vi "StringToCoreArray.vi"(11 "Error In":errorcluster) -> (4 "Key Value Variant":variant, 15 "Error Out":errorcluster)   [LabVIEW 2016, in "Drona.lvlib" / "KeyboardSimulation.lvlib"]
doc: "Gives the key value pair variant output, for various letters present in keyboard"
uses:
  KeyboardSimulation.lvlib
  typedef/VirtualKey.ctl
  typedef/Action.ctl
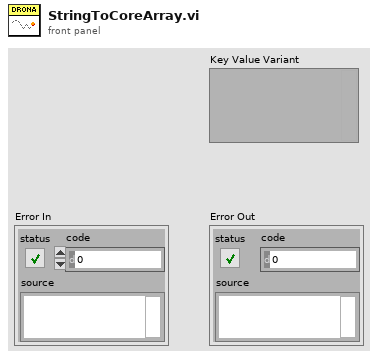
[diagram p1: front panel]
types:
  T1 = typedef "Drona.lvlib/KeyboardSimulation.lvlib/VirtualKey.ctl" = u8
  T2 = typedef "Drona.lvlib/KeyboardSimulation.lvlib/Action.ctl" = enum16{"Press", "Up", "Down"}
  T3 = cluster{"Key":T1, "Action":T2, "Delay (ms)":u32}[]
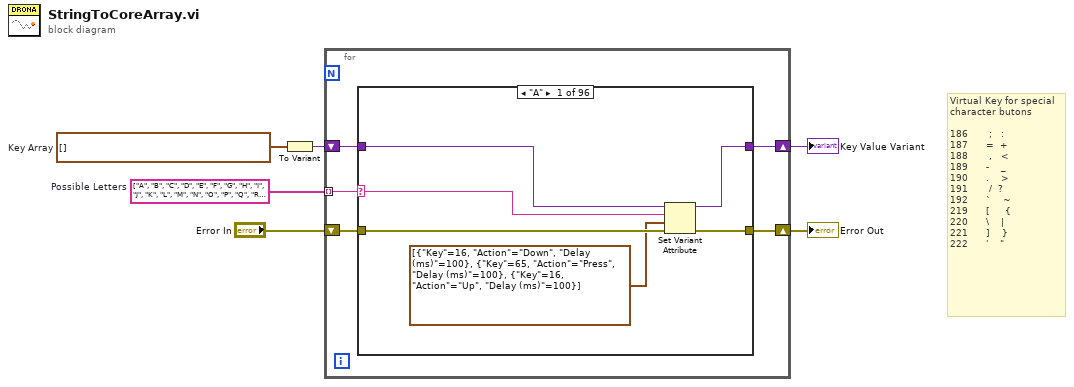
[diagram p0: block diagram]
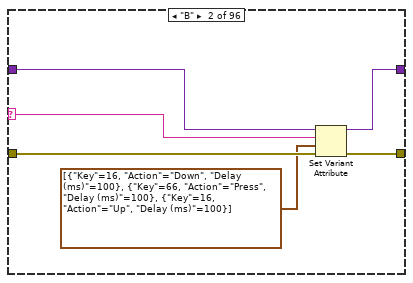
[diagram p2: hidden frame]
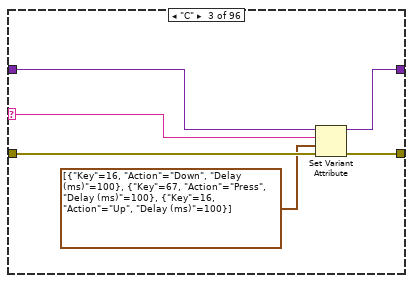
[diagram p3: hidden frame]
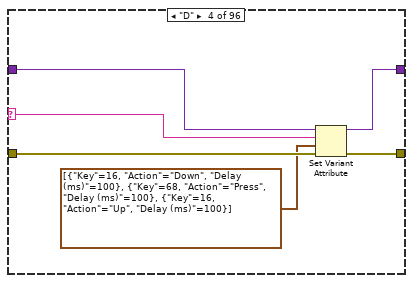
[diagram p4: hidden frame]
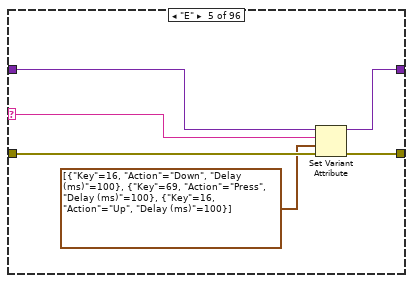
[diagram p5: hidden frame]
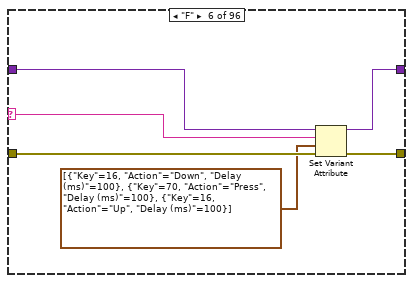
[diagram p6: hidden frame]
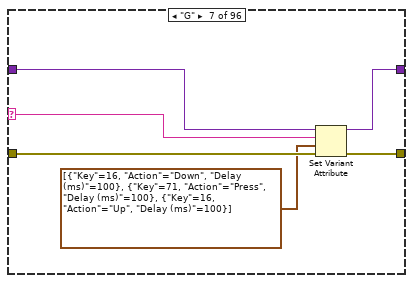
[diagram p7: hidden frame]
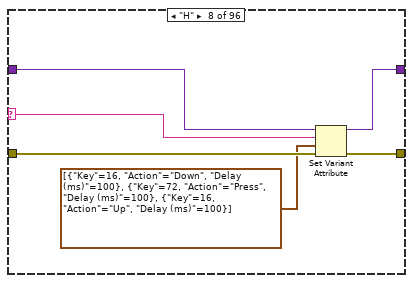
[diagram p8: hidden frame]
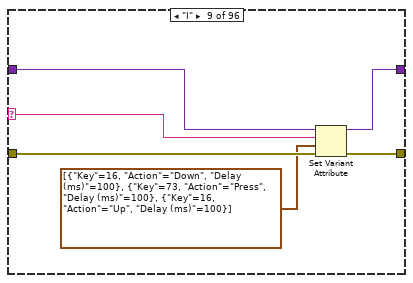
[diagram p9: hidden frame]
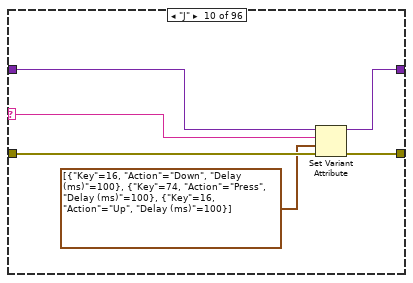
[diagram p10: hidden frame]
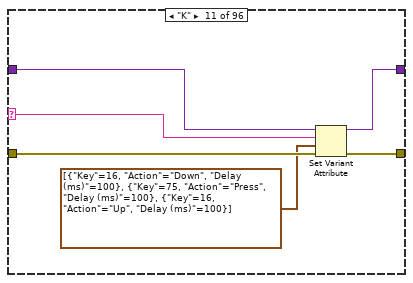
[diagram p11: hidden frame]
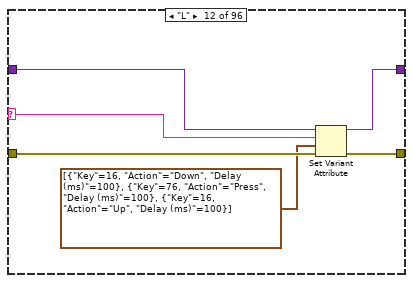
[diagram p12: hidden frame]
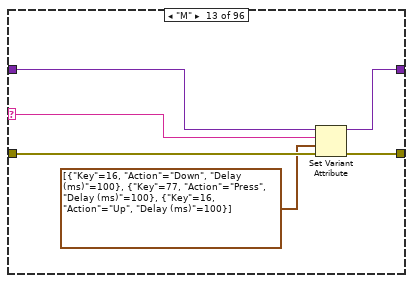
[diagram p13: hidden frame]
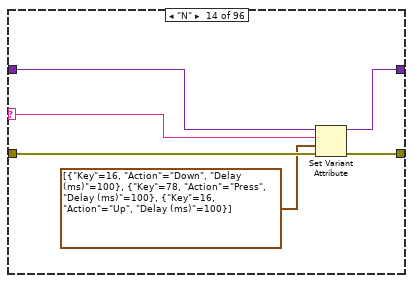
[diagram p14: hidden frame]
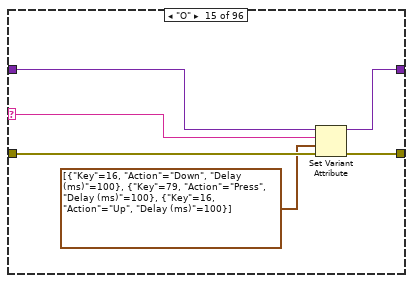
[diagram p15: hidden frame]
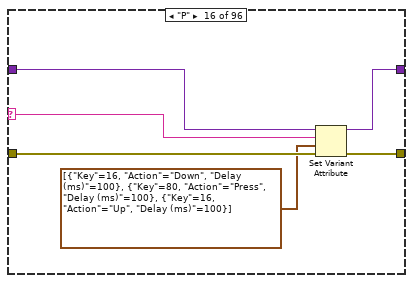
[diagram p16: hidden frame]
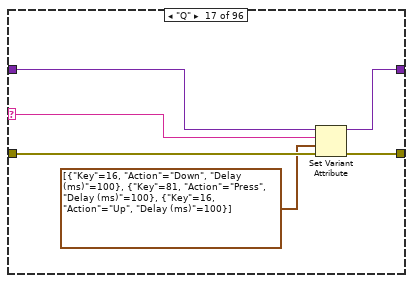
[diagram p17: hidden frame]
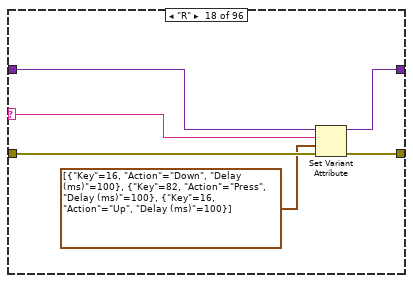
[diagram p18: hidden frame]
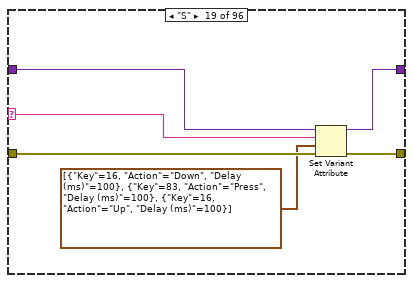
[diagram p19: hidden frame]
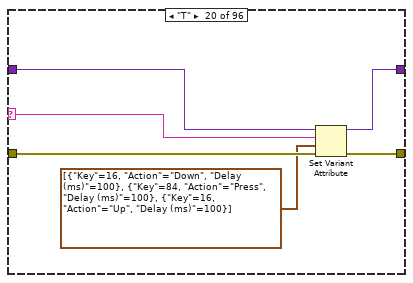
[diagram p20: hidden frame]
diagram:
  w4 = T3 []  # Key Array
  w5 = string[] ["A", "B", "C", "D", "E", "F", "G", "H", "I", "J", "K", "L", "M", "N", "O", "P", "Q", "R", "S", "T", "U", "V", "W", "X", "Y", "Z", "a", "b", "c", "d", "e", "f", "g", "h", "i", "j", "k", "l", "m", "n", "o", "p", "q", "r", "s", "t", "u", "v", "w", "x", "y", "z", "1", "2", "3", "4", "5", "6", "7", "8", "9", "0", "!", "@", "#", "$", "%", "^", "&", "*", "(", ")", ";", ":", "=", "+", ",", "<", "-", "_", ".", ">", "/", "?", "`", "~", "[", "{", "Back Slash", "|", "]", "}", "Single Quotes", "Double Quotes", "Space"]  # Possible Letters
  # "Virtual Key for special character butons\n\n186       ;   :\n187      =  +\n188       ,   <\n189      -    _\n190      .    >\n191       /  ?\n192      `    ~\n219      [     {\n220      \\    |\n221      ]    }\n222      '    \""
  n1 = To Variant(anything=w4) -> (Variant=w3:variant)
  n2 = for {
    shift-right: [w7] -> w1
    shift-left: w3 -> [w9]
    shift-right: [w8] -> w2
    shift-left: "Error In" -> [w10]
    tunnel: w5 -> [w11] mode=indexing
    n3 = case shown="\"A\"" w11 {
      selector: w11 -> [w15 w21 w27 w33 w39 w45 w51 w57 w63 w69 w75 w81 w87 w93 w99 w105 w111 w117 w123 w129 w135 w141 w147 w153 w159 w165 w171 w177 w183 w189 w195 w201 w207 w213 w219 w225 w231 w237 w243 w249 w255 w261 w267 w273 w279 w285 w291 w297 w303 w309 w315 w321 w327 w333 w339 w345 w351 w357 w363 w369 w375 w381 w387 w393 w399 w405 w411 w417 w423 w429 w435 w441 w447 w453 w459 w465 w471 w477 w483 w489 w495 w501 w507 w513 w519 w525 w531 w537 _ w549 w555 w561 _ _ _ _]
      tunnel: w10 -> [w17 w23 w29 w35 w41 w47 w53 w59 w65 w71 w77 w83 w89 w95 w101 w107 w113 w119 w125 w131 w137 w143 w149 w155 w161 w167 w173 w179 w185 w191 w197 w203 w209 w215 w221 w227 w233 w239 w245 w251 w257 w263 w269 w275 w281 w287 w293 w299 w305 w311 w317 w323 w329 w335 w341 w347 w353 w359 w365 w371 w377 w383 w389 w395 w401 w407 w413 w419 w425 w431 w437 w443 w449 w455 w461 w467 w473 w479 w485 w491 w497 w503 w509 w515 w521 w527 w533 w539 w545 w551 w557 w563 w569 w575 w581 w582]
      tunnel: w9 -> [w16 w22 w28 w34 w40 w46 w52 w58 w64 w70 w76 w82 w88 w94 w100 w106 w112 w118 w124 w130 w136 w142 w148 w154 w160 w166 w172 w178 w184 w190 w196 w202 w208 w214 w220 w226 w232 w238 w244 w250 w256 w262 w268 w274 w280 w286 w292 w298 w304 w310 w316 w322 w328 w334 w340 w346 w352 w358 w364 w370 w376 w382 w388 w394 w400 w406 w412 w418 w424 w430 w436 w442 w448 w454 w460 w466 w472 w478 w484 w490 w496 w502 w508 w514 w520 w526 w532 w538 w544 w550 w556 w562 w568 w574 w580 w583]
      tunnel: [w14 w20 w26 w32 w38 w44 w50 w56 w62 w68 w74 w80 w86 w92 w98 w104 w110 w116 w122 w128 w134 w140 w146 w152 w158 w164 w170 w176 w182 w188 w194 w200 w206 w212 w218 w224 w230 w236 w242 w248 w254 w260 w266 w272 w278 w284 w290 w296 w302 w308 w314 w320 w326 w332 w338 w344 w350 w356 w362 w368 w374 w380 w386 w392 w398 w404 w410 w416 w422 w428 w434 w440 w446 w452 w458 w464 w470 w476 w482 w488 w494 w500 w506 w512 w518 w524 w530 w536 w543 w548 w554 w560 w567 w573 w579 w582] -> w8
      tunnel: [w13 w19 w25 w31 w37 w43 w49 w55 w61 w67 w73 w79 w85 w91 w97 w103 w109 w115 w121 w127 w133 w139 w145 w151 w157 w163 w169 w175 w181 w187 w193 w199 w205 w211 w217 w223 w229 w235 w241 w247 w253 w259 w265 w271 w277 w283 w289 w295 w301 w307 w313 w319 w325 w331 w337 w343 w349 w355 w361 w367 w373 w379 w385 w391 w397 w403 w409 w415 w421 w427 w433 w439 w445 w451 w457 w463 w469 w475 w481 w487 w493 w499 w505 w511 w517 w523 w529 w535 w542 w547 w553 w559 w566 w572 w578 w583] -> w7
      frame "A" {
        n4 = Set Variant Attribute(Variant=w16, name=w15, value=T3 [{"Key"=16, "Action"=enum."Down", "Delay (ms)"=100}, {"Key"=65, "Action"=enum."Press", "Delay (ms)"=100}, {"Key"=16, "Action"=enum."Up", "Delay (ms)"=100}] ("Key Array"), error in=w17) -> (Variant out=w13:variant, error out=w14:errorcluster)  [unwired: 1 out]
      }
      frame "B" {
        n5 = Set Variant Attribute(Variant=w22, name=w21, value=T3 [{"Key"=16, "Action"=enum."Down", "Delay (ms)"=100}, {"Key"=66, "Action"=enum."Press", "Delay (ms)"=100}, {"Key"=16, "Action"=enum."Up", "Delay (ms)"=100}] ("Key Array"), error in=w23) -> (Variant out=w19:variant, error out=w20:errorcluster)  [unwired: 1 out]
      }
      frame "C" {
        n6 = Set Variant Attribute(Variant=w28, name=w27, value=T3 [{"Key"=16, "Action"=enum."Down", "Delay (ms)"=100}, {"Key"=67, "Action"=enum."Press", "Delay (ms)"=100}, {"Key"=16, "Action"=enum."Up", "Delay (ms)"=100}] ("Key Array"), error in=w29) -> (Variant out=w25:variant, error out=w26:errorcluster)  [unwired: 1 out]
      }
      frame "D" {
        n7 = Set Variant Attribute(Variant=w34, name=w33, value=T3 [{"Key"=16, "Action"=enum."Down", "Delay (ms)"=100}, {"Key"=68, "Action"=enum."Press", "Delay (ms)"=100}, {"Key"=16, "Action"=enum."Up", "Delay (ms)"=100}] ("Key Array"), error in=w35) -> (Variant out=w31:variant, error out=w32:errorcluster)  [unwired: 1 out]
      }
      frame "E" {
        n8 = Set Variant Attribute(Variant=w40, name=w39, value=T3 [{"Key"=16, "Action"=enum."Down", "Delay (ms)"=100}, {"Key"=69, "Action"=enum."Press", "Delay (ms)"=100}, {"Key"=16, "Action"=enum."Up", "Delay (ms)"=100}] ("Key Array"), error in=w41) -> (Variant out=w37:variant, error out=w38:errorcluster)  [unwired: 1 out]
      }
      frame "F" {
        n9 = Set Variant Attribute(Variant=w46, name=w45, value=T3 [{"Key"=16, "Action"=enum."Down", "Delay (ms)"=100}, {"Key"=70, "Action"=enum."Press", "Delay (ms)"=100}, {"Key"=16, "Action"=enum."Up", "Delay (ms)"=100}] ("Key Array"), error in=w47) -> (Variant out=w43:variant, error out=w44:errorcluster)  [unwired: 1 out]
      }
      frame "G" {
        n10 = Set Variant Attribute(Variant=w52, name=w51, value=T3 [{"Key"=16, "Action"=enum."Down", "Delay (ms)"=100}, {"Key"=71, "Action"=enum."Press", "Delay (ms)"=100}, {"Key"=16, "Action"=enum."Up", "Delay (ms)"=100}] ("Key Array"), error in=w53) -> (Variant out=w49:variant, error out=w50:errorcluster)  [unwired: 1 out]
      }
      frame "H" {
        n11 = Set Variant Attribute(Variant=w58, name=w57, value=T3 [{"Key"=16, "Action"=enum."Down", "Delay (ms)"=100}, {"Key"=72, "Action"=enum."Press", "Delay (ms)"=100}, {"Key"=16, "Action"=enum."Up", "Delay (ms)"=100}] ("Key Array"), error in=w59) -> (Variant out=w55:variant, error out=w56:errorcluster)  [unwired: 1 out]
      }
      frame "I" {
        n12 = Set Variant Attribute(Variant=w64, name=w63, value=T3 [{"Key"=16, "Action"=enum."Down", "Delay (ms)"=100}, {"Key"=73, "Action"=enum."Press", "Delay (ms)"=100}, {"Key"=16, "Action"=enum."Up", "Delay (ms)"=100}] ("Key Array"), error in=w65) -> (Variant out=w61:variant, error out=w62:errorcluster)  [unwired: 1 out]
      }
      frame "J" {
        n13 = Set Variant Attribute(Variant=w70, name=w69, value=T3 [{"Key"=16, "Action"=enum."Down", "Delay (ms)"=100}, {"Key"=74, "Action"=enum."Press", "Delay (ms)"=100}, {"Key"=16, "Action"=enum."Up", "Delay (ms)"=100}] ("Key Array"), error in=w71) -> (Variant out=w67:variant, error out=w68:errorcluster)  [unwired: 1 out]
      }
      frame "K" {
        n14 = Set Variant Attribute(Variant=w76, name=w75, value=T3 [{"Key"=16, "Action"=enum."Down", "Delay (ms)"=100}, {"Key"=75, "Action"=enum."Press", "Delay (ms)"=100}, {"Key"=16, "Action"=enum."Up", "Delay (ms)"=100}] ("Key Array"), error in=w77) -> (Variant out=w73:variant, error out=w74:errorcluster)  [unwired: 1 out]
      }
      frame "L" {
        n15 = Set Variant Attribute(Variant=w82, name=w81, value=T3 [{"Key"=16, "Action"=enum."Down", "Delay (ms)"=100}, {"Key"=76, "Action"=enum."Press", "Delay (ms)"=100}, {"Key"=16, "Action"=enum."Up", "Delay (ms)"=100}] ("Key Array"), error in=w83) -> (Variant out=w79:variant, error out=w80:errorcluster)  [unwired: 1 out]
      }
      frame "M" {
        n16 = Set Variant Attribute(Variant=w88, name=w87, value=T3 [{"Key"=16, "Action"=enum."Down", "Delay (ms)"=100}, {"Key"=77, "Action"=enum."Press", "Delay (ms)"=100}, {"Key"=16, "Action"=enum."Up", "Delay (ms)"=100}] ("Key Array"), error in=w89) -> (Variant out=w85:variant, error out=w86:errorcluster)  [unwired: 1 out]
      }
      frame "N" {
        n17 = Set Variant Attribute(Variant=w94, name=w93, value=T3 [{"Key"=16, "Action"=enum."Down", "Delay (ms)"=100}, {"Key"=78, "Action"=enum."Press", "Delay (ms)"=100}, {"Key"=16, "Action"=enum."Up", "Delay (ms)"=100}] ("Key Array"), error in=w95) -> (Variant out=w91:variant, error out=w92:errorcluster)  [unwired: 1 out]
      }
      frame "O" {
        n18 = Set Variant Attribute(Variant=w100, name=w99, value=T3 [{"Key"=16, "Action"=enum."Down", "Delay (ms)"=100}, {"Key"=79, "Action"=enum."Press", "Delay (ms)"=100}, {"Key"=16, "Action"=enum."Up", "Delay (ms)"=100}] ("Key Array"), error in=w101) -> (Variant out=w97:variant, error out=w98:errorcluster)  [unwired: 1 out]
      }
      frame "P" {
        n19 = Set Variant Attribute(Variant=w106, name=w105, value=T3 [{"Key"=16, "Action"=enum."Down", "Delay (ms)"=100}, {"Key"=80, "Action"=enum."Press", "Delay (ms)"=100}, {"Key"=16, "Action"=enum."Up", "Delay (ms)"=100}] ("Key Array"), error in=w107) -> (Variant out=w103:variant, error out=w104:errorcluster)  [unwired: 1 out]
      }
      frame "Q" {
        n20 = Set Variant Attribute(Variant=w112, name=w111, value=T3 [{"Key"=16, "Action"=enum."Down", "Delay (ms)"=100}, {"Key"=81, "Action"=enum."Press", "Delay (ms)"=100}, {"Key"=16, "Action"=enum."Up", "Delay (ms)"=100}] ("Key Array"), error in=w113) -> (Variant out=w109:variant, error out=w110:errorcluster)  [unwired: 1 out]
      }
      frame "R" {
        n21 = Set Variant Attribute(Variant=w118, name=w117, value=T3 [{"Key"=16, "Action"=enum."Down", "Delay (ms)"=100}, {"Key"=82, "Action"=enum."Press", "Delay (ms)"=100}, {"Key"=16, "Action"=enum."Up", "Delay (ms)"=100}] ("Key Array"), error in=w119) -> (Variant out=w115:variant, error out=w116:errorcluster)  [unwired: 1 out]
      }
      frame "S" {
        n22 = Set Variant Attribute(Variant=w124, name=w123, value=T3 [{"Key"=16, "Action"=enum."Down", "Delay (ms)"=100}, {"Key"=83, "Action"=enum."Press", "Delay (ms)"=100}, {"Key"=16, "Action"=enum."Up", "Delay (ms)"=100}] ("Key Array"), error in=w125) -> (Variant out=w121:variant, error out=w122:errorcluster)  [unwired: 1 out]
      }
      frame "T" {
        n23 = Set Variant Attribute(Variant=w130, name=w129, value=T3 [{"Key"=16, "Action"=enum."Down", "Delay (ms)"=100}, {"Key"=84, "Action"=enum."Press", "Delay (ms)"=100}, {"Key"=16, "Action"=enum."Up", "Delay (ms)"=100}] ("Key Array"), error in=w131) -> (Variant out=w127:variant, error out=w128:errorcluster)  [unwired: 1 out]
      }
      frame "U" {
        n24 = Set Variant Attribute(Variant=w136, name=w135, value=T3 [{"Key"=16, "Action"=enum."Down", "Delay (ms)"=100}, {"Key"=85, "Action"=enum."Press", "Delay (ms)"=100}, {"Key"=16, "Action"=enum."Up", "Delay (ms)"=100}] ("Key Array"), error in=w137) -> (Variant out=w133:variant, error out=w134:errorcluster)  [unwired: 1 out]
      }
      frame "V" {
        n25 = Set Variant Attribute(Variant=w142, name=w141, value=T3 [{"Key"=16, "Action"=enum."Down", "Delay (ms)"=100}, {"Key"=86, "Action"=enum."Press", "Delay (ms)"=100}, {"Key"=16, "Action"=enum."Up", "Delay (ms)"=100}] ("Key Array"), error in=w143) -> (Variant out=w139:variant, error out=w140:errorcluster)  [unwired: 1 out]
      }
      frame "W" {
        n26 = Set Variant Attribute(Variant=w148, name=w147, value=T3 [{"Key"=16, "Action"=enum."Down", "Delay (ms)"=100}, {"Key"=87, "Action"=enum."Press", "Delay (ms)"=100}, {"Key"=16, "Action"=enum."Up", "Delay (ms)"=100}] ("Key Array"), error in=w149) -> (Variant out=w145:variant, error out=w146:errorcluster)  [unwired: 1 out]
      }
      frame "X" {
        n27 = Set Variant Attribute(Variant=w154, name=w153, value=T3 [{"Key"=16, "Action"=enum."Down", "Delay (ms)"=100}, {"Key"=88, "Action"=enum."Press", "Delay (ms)"=100}, {"Key"=16, "Action"=enum."Up", "Delay (ms)"=100}] ("Key Array"), error in=w155) -> (Variant out=w151:variant, error out=w152:errorcluster)  [unwired: 1 out]
      }
      frame "Y" {
        n28 = Set Variant Attribute(Variant=w160, name=w159, value=T3 [{"Key"=16, "Action"=enum."Down", "Delay (ms)"=100}, {"Key"=89, "Action"=enum."Press", "Delay (ms)"=100}, {"Key"=16, "Action"=enum."Up", "Delay (ms)"=100}] ("Key Array"), error in=w161) -> (Variant out=w157:variant, error out=w158:errorcluster)  [unwired: 1 out]
      }
      frame "Z" {
        n29 = Set Variant Attribute(Variant=w166, name=w165, value=T3 [{"Key"=16, "Action"=enum."Down", "Delay (ms)"=100}, {"Key"=90, "Action"=enum."Press", "Delay (ms)"=100}, {"Key"=16, "Action"=enum."Up", "Delay (ms)"=100}] ("Key Array"), error in=w167) -> (Variant out=w163:variant, error out=w164:errorcluster)  [unwired: 1 out]
      }
      frame "a" {
        n30 = Set Variant Attribute(Variant=w172, name=w171, value=T3 [{"Key"=65, "Action"=enum."Press", "Delay (ms)"=100}] ("Key Array"), error in=w173) -> (Variant out=w169:variant, error out=w170:errorcluster)  [unwired: 1 out]
      }
      frame "b" {
        n31 = Set Variant Attribute(Variant=w178, name=w177, value=T3 [{"Key"=66, "Action"=enum."Press", "Delay (ms)"=100}] ("Key Array"), error in=w179) -> (Variant out=w175:variant, error out=w176:errorcluster)  [unwired: 1 out]
      }
      frame "c" {
        n32 = Set Variant Attribute(Variant=w184, name=w183, value=T3 [{"Key"=67, "Action"=enum."Press", "Delay (ms)"=100}] ("Key Array"), error in=w185) -> (Variant out=w181:variant, error out=w182:errorcluster)  [unwired: 1 out]
      }
      frame "d" {
        n33 = Set Variant Attribute(Variant=w190, name=w189, value=T3 [{"Key"=68, "Action"=enum."Press", "Delay (ms)"=100}] ("Key Array"), error in=w191) -> (Variant out=w187:variant, error out=w188:errorcluster)  [unwired: 1 out]
      }
      frame "e" {
        n34 = Set Variant Attribute(Variant=w196, name=w195, value=T3 [{"Key"=69, "Action"=enum."Press", "Delay (ms)"=100}] ("Key Array"), error in=w197) -> (Variant out=w193:variant, error out=w194:errorcluster)  [unwired: 1 out]
      }
      frame "f" {
        n35 = Set Variant Attribute(Variant=w202, name=w201, value=T3 [{"Key"=70, "Action"=enum."Press", "Delay (ms)"=100}] ("Key Array"), error in=w203) -> (Variant out=w199:variant, error out=w200:errorcluster)  [unwired: 1 out]
      }
      frame "g" {
        n36 = Set Variant Attribute(Variant=w208, name=w207, value=T3 [{"Key"=71, "Action"=enum."Press", "Delay (ms)"=100}] ("Key Array"), error in=w209) -> (Variant out=w205:variant, error out=w206:errorcluster)  [unwired: 1 out]
      }
      frame "h" {
        n37 = Set Variant Attribute(Variant=w214, name=w213, value=T3 [{"Key"=72, "Action"=enum."Press", "Delay (ms)"=100}] ("Key Array"), error in=w215) -> (Variant out=w211:variant, error out=w212:errorcluster)  [unwired: 1 out]
      }
      frame "i" {
        n38 = Set Variant Attribute(Variant=w220, name=w219, value=T3 [{"Key"=73, "Action"=enum."Press", "Delay (ms)"=100}] ("Key Array"), error in=w221) -> (Variant out=w217:variant, error out=w218:errorcluster)  [unwired: 1 out]
      }
      frame "j" {
        n39 = Set Variant Attribute(Variant=w226, name=w225, value=T3 [{"Key"=74, "Action"=enum."Press", "Delay (ms)"=100}] ("Key Array"), error in=w227) -> (Variant out=w223:variant, error out=w224:errorcluster)  [unwired: 1 out]
      }
      frame "k" {
        n40 = Set Variant Attribute(Variant=w232, name=w231, value=T3 [{"Key"=75, "Action"=enum."Press", "Delay (ms)"=100}] ("Key Array"), error in=w233) -> (Variant out=w229:variant, error out=w230:errorcluster)  [unwired: 1 out]
      }
      frame "l" {
        n41 = Set Variant Attribute(Variant=w238, name=w237, value=T3 [{"Key"=76, "Action"=enum."Press", "Delay (ms)"=100}] ("Key Array"), error in=w239) -> (Variant out=w235:variant, error out=w236:errorcluster)  [unwired: 1 out]
      }
      frame "m" {
        n42 = Set Variant Attribute(Variant=w244, name=w243, value=T3 [{"Key"=77, "Action"=enum."Press", "Delay (ms)"=100}] ("Key Array"), error in=w245) -> (Variant out=w241:variant, error out=w242:errorcluster)  [unwired: 1 out]
      }
      frame "n" {
        n43 = Set Variant Attribute(Variant=w250, name=w249, value=T3 [{"Key"=78, "Action"=enum."Press", "Delay (ms)"=100}] ("Key Array"), error in=w251) -> (Variant out=w247:variant, error out=w248:errorcluster)  [unwired: 1 out]
      }
      frame "o" {
        n44 = Set Variant Attribute(Variant=w256, name=w255, value=T3 [{"Key"=79, "Action"=enum."Press", "Delay (ms)"=100}] ("Key Array"), error in=w257) -> (Variant out=w253:variant, error out=w254:errorcluster)  [unwired: 1 out]
      }
      frame "p" {
        n45 = Set Variant Attribute(Variant=w262, name=w261, value=T3 [{"Key"=80, "Action"=enum."Press", "Delay (ms)"=100}] ("Key Array"), error in=w263) -> (Variant out=w259:variant, error out=w260:errorcluster)  [unwired: 1 out]
      }
      frame "q" {
        n46 = Set Variant Attribute(Variant=w268, name=w267, value=T3 [{"Key"=81, "Action"=enum."Press", "Delay (ms)"=100}] ("Key Array"), error in=w269) -> (Variant out=w265:variant, error out=w266:errorcluster)  [unwired: 1 out]
      }
      frame "r" {
        n47 = Set Variant Attribute(Variant=w274, name=w273, value=T3 [{"Key"=82, "Action"=enum."Press", "Delay (ms)"=100}] ("Key Array"), error in=w275) -> (Variant out=w271:variant, error out=w272:errorcluster)  [unwired: 1 out]
      }
      frame "s" {
        n48 = Set Variant Attribute(Variant=w280, name=w279, value=T3 [{"Key"=83, "Action"=enum."Press", "Delay (ms)"=100}] ("Key Array"), error in=w281) -> (Variant out=w277:variant, error out=w278:errorcluster)  [unwired: 1 out]
      }
      frame "t" {
        n49 = Set Variant Attribute(Variant=w286, name=w285, value=T3 [{"Key"=84, "Action"=enum."Press", "Delay (ms)"=100}] ("Key Array"), error in=w287) -> (Variant out=w283:variant, error out=w284:errorcluster)  [unwired: 1 out]
      }
      frame "u" {
        n50 = Set Variant Attribute(Variant=w292, name=w291, value=T3 [{"Key"=85, "Action"=enum."Press", "Delay (ms)"=100}] ("Key Array"), error in=w293) -> (Variant out=w289:variant, error out=w290:errorcluster)  [unwired: 1 out]
      }
      frame "v" {
        n51 = Set Variant Attribute(Variant=w298, name=w297, value=T3 [{"Key"=86, "Action"=enum."Press", "Delay (ms)"=100}] ("Key Array"), error in=w299) -> (Variant out=w295:variant, error out=w296:errorcluster)  [unwired: 1 out]
      }
      frame "w" {
        n52 = Set Variant Attribute(Variant=w304, name=w303, value=T3 [{"Key"=87, "Action"=enum."Press", "Delay (ms)"=100}] ("Key Array"), error in=w305) -> (Variant out=w301:variant, error out=w302:errorcluster)  [unwired: 1 out]
      }
      frame "x" {
        n53 = Set Variant Attribute(Variant=w310, name=w309, value=T3 [{"Key"=88, "Action"=enum."Press", "Delay (ms)"=100}] ("Key Array"), error in=w311) -> (Variant out=w307:variant, error out=w308:errorcluster)  [unwired: 1 out]
      }
      frame "y" {
        n54 = Set Variant Attribute(Variant=w316, name=w315, value=T3 [{"Key"=89, "Action"=enum."Press", "Delay (ms)"=100}] ("Key Array"), error in=w317) -> (Variant out=w313:variant, error out=w314:errorcluster)  [unwired: 1 out]
      }
      frame "z" {
        n55 = Set Variant Attribute(Variant=w322, name=w321, value=T3 [{"Key"=90, "Action"=enum."Press", "Delay (ms)"=100}] ("Key Array"), error in=w323) -> (Variant out=w319:variant, error out=w320:errorcluster)  [unwired: 1 out]
      }
      frame "1" {
        n56 = Set Variant Attribute(Variant=w328, name=w327, value=T3 [{"Key"=49, "Action"=enum."Press", "Delay (ms)"=100}] ("Key Array"), error in=w329) -> (Variant out=w325:variant, error out=w326:errorcluster)  [unwired: 1 out]
      }
      frame "2" {
        n57 = Set Variant Attribute(Variant=w334, name=w333, value=T3 [{"Key"=50, "Action"=enum."Press", "Delay (ms)"=100}] ("Key Array"), error in=w335) -> (Variant out=w331:variant, error out=w332:errorcluster)  [unwired: 1 out]
      }
      frame "3" {
        n58 = Set Variant Attribute(Variant=w340, name=w339, value=T3 [{"Key"=51, "Action"=enum."Press", "Delay (ms)"=100}] ("Key Array"), error in=w341) -> (Variant out=w337:variant, error out=w338:errorcluster)  [unwired: 1 out]
      }
      frame "4" {
        n59 = Set Variant Attribute(Variant=w346, name=w345, value=T3 [{"Key"=52, "Action"=enum."Press", "Delay (ms)"=100}] ("Key Array"), error in=w347) -> (Variant out=w343:variant, error out=w344:errorcluster)  [unwired: 1 out]
      }
      frame "5" {
        n60 = Set Variant Attribute(Variant=w352, name=w351, value=T3 [{"Key"=53, "Action"=enum."Press", "Delay (ms)"=100}] ("Key Array"), error in=w353) -> (Variant out=w349:variant, error out=w350:errorcluster)  [unwired: 1 out]
      }
      frame "6" {
        n61 = Set Variant Attribute(Variant=w358, name=w357, value=T3 [{"Key"=54, "Action"=enum."Press", "Delay (ms)"=100}] ("Key Array"), error in=w359) -> (Variant out=w355:variant, error out=w356:errorcluster)  [unwired: 1 out]
      }
      frame "7" {
        n62 = Set Variant Attribute(Variant=w364, name=w363, value=T3 [{"Key"=55, "Action"=enum."Press", "Delay (ms)"=100}] ("Key Array"), error in=w365) -> (Variant out=w361:variant, error out=w362:errorcluster)  [unwired: 1 out]
      }
      frame "8" {
        n63 = Set Variant Attribute(Variant=w370, name=w369, value=T3 [{"Key"=56, "Action"=enum."Press", "Delay (ms)"=100}] ("Key Array"), error in=w371) -> (Variant out=w367:variant, error out=w368:errorcluster)  [unwired: 1 out]
      }
      frame "9" {
        n64 = Set Variant Attribute(Variant=w376, name=w375, value=T3 [{"Key"=57, "Action"=enum."Press", "Delay (ms)"=100}] ("Key Array"), error in=w377) -> (Variant out=w373:variant, error out=w374:errorcluster)  [unwired: 1 out]
      }
      frame "0" {
        n65 = Set Variant Attribute(Variant=w382, name=w381, value=T3 [{"Key"=48, "Action"=enum."Press", "Delay (ms)"=100}] ("Key Array"), error in=w383) -> (Variant out=w379:variant, error out=w380:errorcluster)  [unwired: 1 out]
      }
      frame "!" {
        n66 = Set Variant Attribute(Variant=w388, name=w387, value=T3 [{"Key"=16, "Action"=enum."Down", "Delay (ms)"=100}, {"Key"=49, "Action"=enum."Press", "Delay (ms)"=100}, {"Key"=16, "Action"=enum."Up", "Delay (ms)"=100}] ("Key Array"), error in=w389) -> (Variant out=w385:variant, error out=w386:errorcluster)  [unwired: 1 out]
      }
      frame "@" {
        n67 = Set Variant Attribute(Variant=w394, name=w393, value=T3 [{"Key"=16, "Action"=enum."Down", "Delay (ms)"=100}, {"Key"=50, "Action"=enum."Press", "Delay (ms)"=100}, {"Key"=16, "Action"=enum."Up", "Delay (ms)"=100}] ("Key Array"), error in=w395) -> (Variant out=w391:variant, error out=w392:errorcluster)  [unwired: 1 out]
      }
      frame "#" {
        n68 = Set Variant Attribute(Variant=w400, name=w399, value=T3 [{"Key"=16, "Action"=enum."Down", "Delay (ms)"=100}, {"Key"=51, "Action"=enum."Press", "Delay (ms)"=100}, {"Key"=16, "Action"=enum."Up", "Delay (ms)"=100}] ("Key Array"), error in=w401) -> (Variant out=w397:variant, error out=w398:errorcluster)  [unwired: 1 out]
      }
      frame "$" {
        n69 = Set Variant Attribute(Variant=w406, name=w405, value=T3 [{"Key"=16, "Action"=enum."Down", "Delay (ms)"=100}, {"Key"=52, "Action"=enum."Press", "Delay (ms)"=100}, {"Key"=16, "Action"=enum."Up", "Delay (ms)"=100}] ("Key Array"), error in=w407) -> (Variant out=w403:variant, error out=w404:errorcluster)  [unwired: 1 out]
      }
      frame "%" {
        n70 = Set Variant Attribute(Variant=w412, name=w411, value=T3 [{"Key"=16, "Action"=enum."Down", "Delay (ms)"=100}, {"Key"=53, "Action"=enum."Press", "Delay (ms)"=100}, {"Key"=16, "Action"=enum."Up", "Delay (ms)"=100}] ("Key Array"), error in=w413) -> (Variant out=w409:variant, error out=w410:errorcluster)  [unwired: 1 out]
      }
      frame "^" {
        n71 = Set Variant Attribute(Variant=w418, name=w417, value=T3 [{"Key"=16, "Action"=enum."Down", "Delay (ms)"=100}, {"Key"=54, "Action"=enum."Press", "Delay (ms)"=100}, {"Key"=16, "Action"=enum."Up", "Delay (ms)"=100}] ("Key Array"), error in=w419) -> (Variant out=w415:variant, error out=w416:errorcluster)  [unwired: 1 out]
      }
      frame "&" {
        n72 = Set Variant Attribute(Variant=w424, name=w423, value=T3 [{"Key"=16, "Action"=enum."Down", "Delay (ms)"=100}, {"Key"=55, "Action"=enum."Press", "Delay (ms)"=100}, {"Key"=16, "Action"=enum."Up", "Delay (ms)"=100}] ("Key Array"), error in=w425) -> (Variant out=w421:variant, error out=w422:errorcluster)  [unwired: 1 out]
      }
      frame "*" {
        n73 = Set Variant Attribute(Variant=w430, name=w429, value=T3 [{"Key"=16, "Action"=enum."Down", "Delay (ms)"=100}, {"Key"=56, "Action"=enum."Press", "Delay (ms)"=100}, {"Key"=16, "Action"=enum."Up", "Delay (ms)"=100}] ("Key Array"), error in=w431) -> (Variant out=w427:variant, error out=w428:errorcluster)  [unwired: 1 out]
      }
      frame "(" {
        n74 = Set Variant Attribute(Variant=w436, name=w435, value=T3 [{"Key"=16, "Action"=enum."Down", "Delay (ms)"=100}, {"Key"=57, "Action"=enum."Press", "Delay (ms)"=100}, {"Key"=16, "Action"=enum."Up", "Delay (ms)"=100}] ("Key Array"), error in=w437) -> (Variant out=w433:variant, error out=w434:errorcluster)  [unwired: 1 out]
      }
      frame ")" {
        n75 = Set Variant Attribute(Variant=w442, name=w441, value=T3 [{"Key"=16, "Action"=enum."Down", "Delay (ms)"=100}, {"Key"=48, "Action"=enum."Press", "Delay (ms)"=100}, {"Key"=16, "Action"=enum."Up", "Delay (ms)"=100}] ("Key Array"), error in=w443) -> (Variant out=w439:variant, error out=w440:errorcluster)  [unwired: 1 out]
      }
      frame ";" {
        n76 = Set Variant Attribute(Variant=w448, name=w447, value=T3 [{"Key"=186, "Action"=enum."Press", "Delay (ms)"=100}] ("Key Array"), error in=w449) -> (Variant out=w445:variant, error out=w446:errorcluster)  [unwired: 1 out]
      }
      frame ":" {
        n77 = Set Variant Attribute(Variant=w454, name=w453, value=T3 [{"Key"=16, "Action"=enum."Down", "Delay (ms)"=100}, {"Key"=186, "Action"=enum."Press", "Delay (ms)"=100}, {"Key"=16, "Action"=enum."Up", "Delay (ms)"=100}] ("Key Array"), error in=w455) -> (Variant out=w451:variant, error out=w452:errorcluster)  [unwired: 1 out]
      }
      frame "=" {
        n78 = Set Variant Attribute(Variant=w460, name=w459, value=T3 [{"Key"=187, "Action"=enum."Press", "Delay (ms)"=100}] ("Key Array"), error in=w461) -> (Variant out=w457:variant, error out=w458:errorcluster)  [unwired: 1 out]
      }
      frame "+" {
        n79 = Set Variant Attribute(Variant=w466, name=w465, value=T3 [{"Key"=16, "Action"=enum."Down", "Delay (ms)"=100}, {"Key"=187, "Action"=enum."Press", "Delay (ms)"=100}, {"Key"=16, "Action"=enum."Up", "Delay (ms)"=100}] ("Key Array"), error in=w467) -> (Variant out=w463:variant, error out=w464:errorcluster)  [unwired: 1 out]
      }
      frame "," {
        n80 = Set Variant Attribute(Variant=w472, name=w471, value=T3 [{"Key"=188, "Action"=enum."Press", "Delay (ms)"=100}] ("Key Array"), error in=w473) -> (Variant out=w469:variant, error out=w470:errorcluster)  [unwired: 1 out]
      }
      frame "<" {
        n81 = Set Variant Attribute(Variant=w478, name=w477, value=T3 [{"Key"=16, "Action"=enum."Down", "Delay (ms)"=100}, {"Key"=188, "Action"=enum."Press", "Delay (ms)"=100}, {"Key"=16, "Action"=enum."Up", "Delay (ms)"=100}] ("Key Array"), error in=w479) -> (Variant out=w475:variant, error out=w476:errorcluster)  [unwired: 1 out]
      }
      frame "-" {
        n82 = Set Variant Attribute(Variant=w484, name=w483, value=T3 [{"Key"=189, "Action"=enum."Press", "Delay (ms)"=100}] ("Key Array"), error in=w485) -> (Variant out=w481:variant, error out=w482:errorcluster)  [unwired: 1 out]
      }
      frame "_" {
        n83 = Set Variant Attribute(Variant=w490, name=w489, value=T3 [{"Key"=16, "Action"=enum."Down", "Delay (ms)"=100}, {"Key"=189, "Action"=enum."Press", "Delay (ms)"=100}, {"Key"=16, "Action"=enum."Up", "Delay (ms)"=100}] ("Key Array"), error in=w491) -> (Variant out=w487:variant, error out=w488:errorcluster)  [unwired: 1 out]
      }
      frame "." {
        n84 = Set Variant Attribute(Variant=w496, name=w495, value=T3 [{"Key"=190, "Action"=enum."Press", "Delay (ms)"=100}] ("Key Array"), error in=w497) -> (Variant out=w493:variant, error out=w494:errorcluster)  [unwired: 1 out]
      }
      frame ">" {
        n85 = Set Variant Attribute(Variant=w502, name=w501, value=T3 [{"Key"=16, "Action"=enum."Down", "Delay (ms)"=100}, {"Key"=190, "Action"=enum."Press", "Delay (ms)"=100}, {"Key"=16, "Action"=enum."Up", "Delay (ms)"=100}] ("Key Array"), error in=w503) -> (Variant out=w499:variant, error out=w500:errorcluster)  [unwired: 1 out]
      }
      frame "/" {
        n86 = Set Variant Attribute(Variant=w508, name=w507, value=T3 [{"Key"=191, "Action"=enum."Press", "Delay (ms)"=100}] ("Key Array"), error in=w509) -> (Variant out=w505:variant, error out=w506:errorcluster)  [unwired: 1 out]
      }
      frame "?" {
        n87 = Set Variant Attribute(Variant=w514, name=w513, value=T3 [{"Key"=16, "Action"=enum."Down", "Delay (ms)"=100}, {"Key"=191, "Action"=enum."Press", "Delay (ms)"=100}, {"Key"=16, "Action"=enum."Up", "Delay (ms)"=100}] ("Key Array"), error in=w515) -> (Variant out=w511:variant, error out=w512:errorcluster)  [unwired: 1 out]
      }
      frame "`" {
        n88 = Set Variant Attribute(Variant=w520, name=w519, value=T3 [{"Key"=192, "Action"=enum."Press", "Delay (ms)"=100}] ("Key Array"), error in=w521) -> (Variant out=w517:variant, error out=w518:errorcluster)  [unwired: 1 out]
      }
      frame "~" {
        n89 = Set Variant Attribute(Variant=w526, name=w525, value=T3 [{"Key"=16, "Action"=enum."Down", "Delay (ms)"=100}, {"Key"=192, "Action"=enum."Press", "Delay (ms)"=100}, {"Key"=16, "Action"=enum."Up", "Delay (ms)"=100}] ("Key Array"), error in=w527) -> (Variant out=w523:variant, error out=w524:errorcluster)  [unwired: 1 out]
      }
      frame "[" {
        n90 = Set Variant Attribute(Variant=w532, name=w531, value=T3 [{"Key"=219, "Action"=enum."Press", "Delay (ms)"=100}] ("Key Array"), error in=w533) -> (Variant out=w529:variant, error out=w530:errorcluster)  [unwired: 1 out]
      }
      frame "{" {
        n91 = Set Variant Attribute(Variant=w538, name=w537, value=T3 [{"Key"=16, "Action"=enum."Down", "Delay (ms)"=100}, {"Key"=219, "Action"=enum."Press", "Delay (ms)"=100}, {"Key"=16, "Action"=enum."Up", "Delay (ms)"=100}] ("Key Array"), error in=w539) -> (Variant out=w535:variant, error out=w536:errorcluster)  [unwired: 1 out]
      }
      frame "Back Slash" {
        n92 = Set Variant Attribute(Variant=w544, name="\\", value=T3 [{"Key"=220, "Action"=enum."Press", "Delay (ms)"=100}] ("Key Array"), error in=w545) -> (Variant out=w542:variant, error out=w543:errorcluster)  [unwired: 1 out]
      }
      frame "|" {
        n93 = Set Variant Attribute(Variant=w550, name=w549, value=T3 [{"Key"=16, "Action"=enum."Down", "Delay (ms)"=100}, {"Key"=220, "Action"=enum."Press", "Delay (ms)"=100}, {"Key"=16, "Action"=enum."Up", "Delay (ms)"=100}] ("Key Array"), error in=w551) -> (Variant out=w547:variant, error out=w548:errorcluster)  [unwired: 1 out]
      }
      frame "]" {
        n94 = Set Variant Attribute(Variant=w556, name=w555, value=T3 [{"Key"=221, "Action"=enum."Press", "Delay (ms)"=100}] ("Key Array"), error in=w557) -> (Variant out=w553:variant, error out=w554:errorcluster)  [unwired: 1 out]
      }
      frame "}" {
        n95 = Set Variant Attribute(Variant=w562, name=w561, value=T3 [{"Key"=16, "Action"=enum."Down", "Delay (ms)"=100}, {"Key"=221, "Action"=enum."Press", "Delay (ms)"=100}, {"Key"=16, "Action"=enum."Up", "Delay (ms)"=100}] ("Key Array"), error in=w563) -> (Variant out=w559:variant, error out=w560:errorcluster)  [unwired: 1 out]
      }
      frame "Single Quotes" {
        n96 = Set Variant Attribute(Variant=w568, name="'", value=T3 [{"Key"=222, "Action"=enum."Press", "Delay (ms)"=100}] ("Key Array"), error in=w569) -> (Variant out=w566:variant, error out=w567:errorcluster)  [unwired: 1 out]
      }
      frame "Double Quotes" {
        n97 = Set Variant Attribute(Variant=w574, name="\"", value=T3 [{"Key"=16, "Action"=enum."Down", "Delay (ms)"=100}, {"Key"=222, "Action"=enum."Press", "Delay (ms)"=100}, {"Key"=16, "Action"=enum."Up", "Delay (ms)"=100}] ("Key Array"), error in=w575) -> (Variant out=w572:variant, error out=w573:errorcluster)  [unwired: 1 out]
      }
      frame "Space" {
        n98 = call <vilib>:"Space Constant.vi"() -> ("String"=w576:string)
        n99 = Set Variant Attribute(Variant=w580, name=w576, value=T3 [{"Key"=32, "Action"=enum."Press", "Delay (ms)"=100}] ("Key Array"), error in=w581) -> (Variant out=w578:variant, error out=w579:errorcluster)  [unwired: 1 out]
      }
      frame Default {
      }
    }
  }
  "Error Out" <- w2
  "Key Value Variant" <- w1
